vi "ReadSlotsNode.vi"(8 "Error In":errorcluster, 11 "Multiplexer Node In":refnum<k20>) -> (0 "Error Out":errorcluster, 2 "Slots":T1[](array[typedef]), 3 "Multiplexer Node Out":refnum<k20>)   [LabVIEW 2012]
uses:
  SlotConfiguration.ctl
  BankConfiguration.ctl
  <vilib>/xml/NI_XML.lvlib
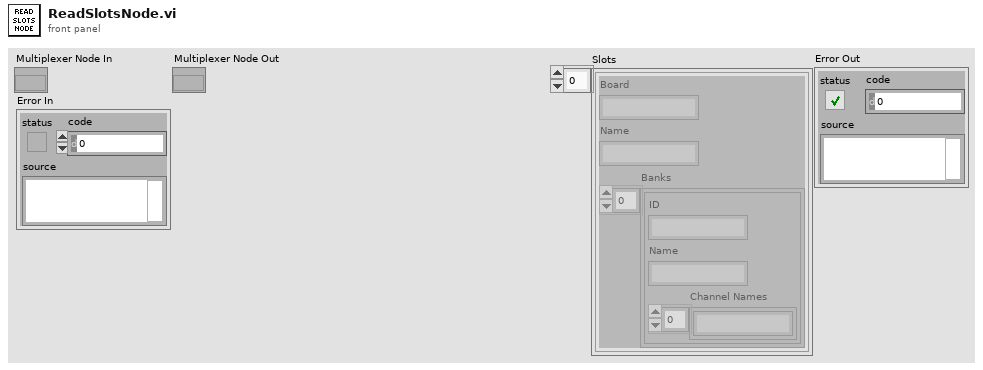
[diagram p1: front panel]
types:
  T1 = typedef "SlotConfiguration.ctl" = cluster{"Board":string, "Name":string, "Banks":T2[]}
  T2 = typedef "BankConfiguration.ctl" = cluster{"ID":string, "Name":string, "Channel Names":string[]}
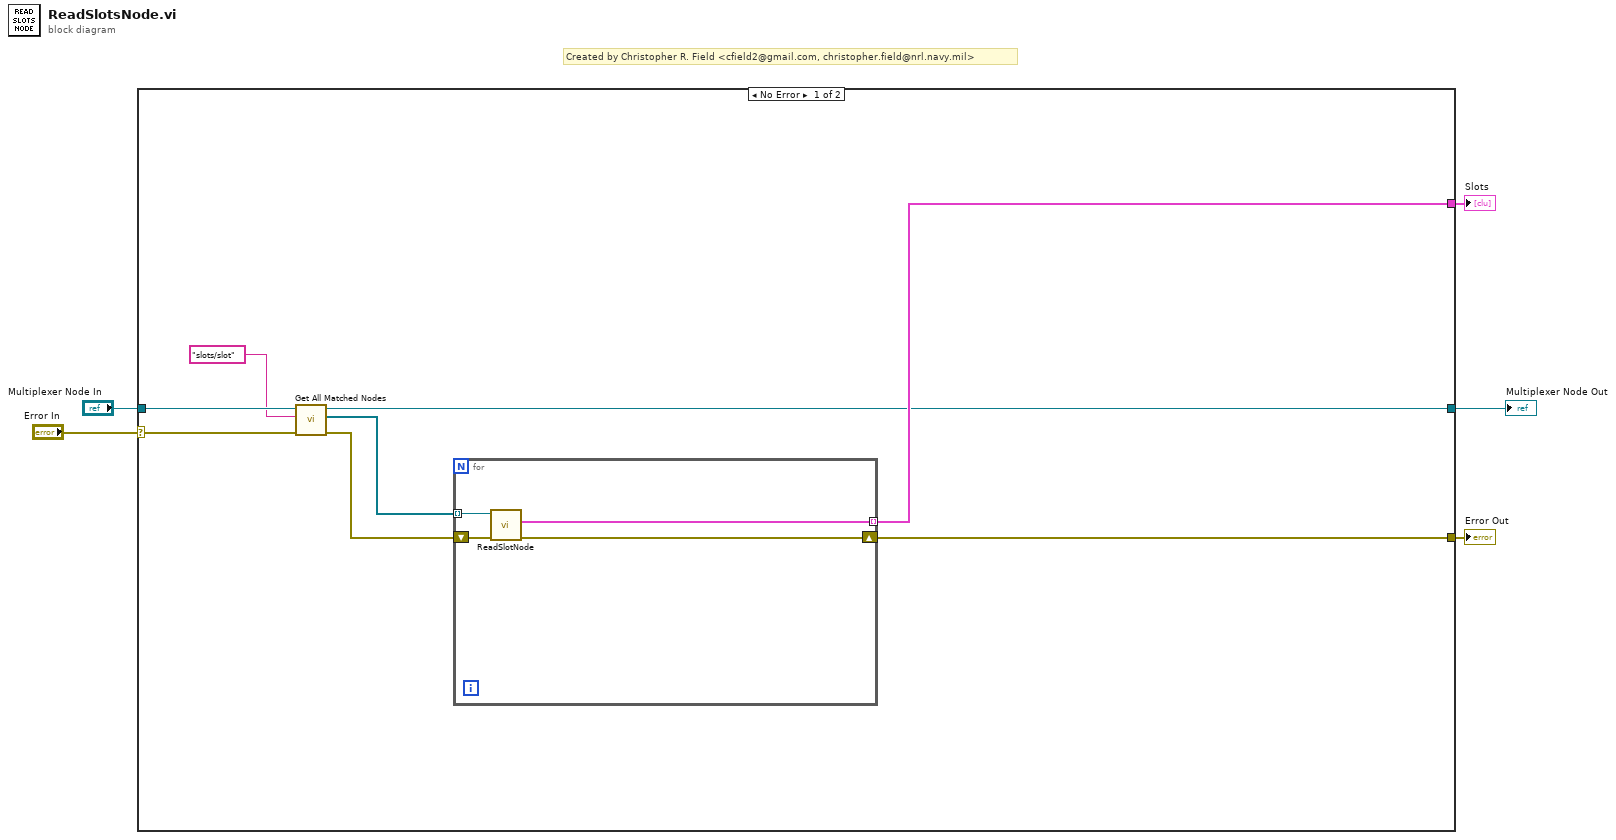
[diagram p0: block diagram]
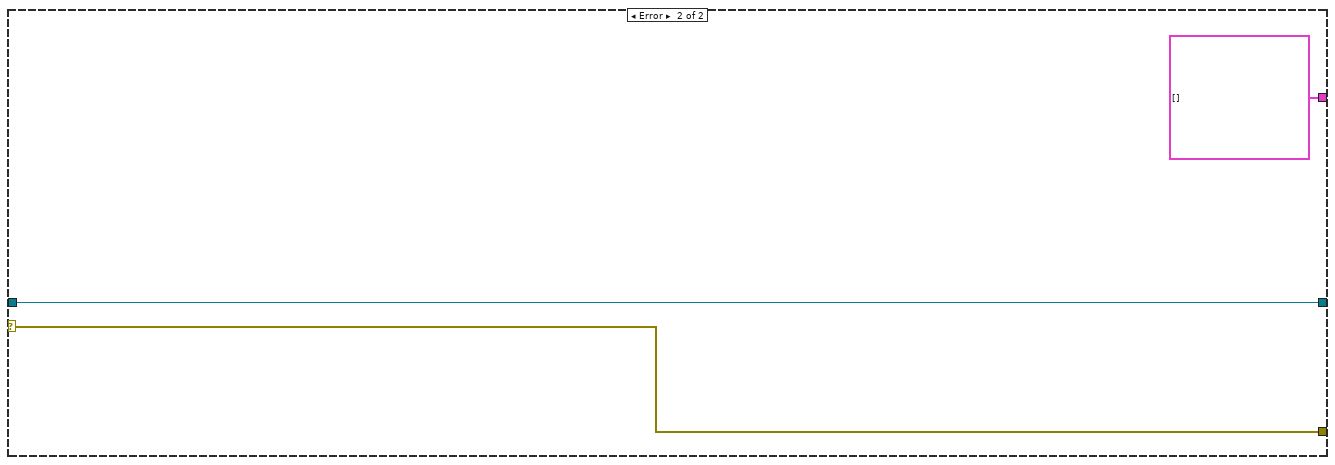
[diagram p2: hidden frame]
diagram:
  # "Created by Christopher R. Field <cfield2@gmail.com, christopher.field@nrl.navy.mil>"
  n1 = case shown="No Error" "Error In" {
    selector: "Error In" -> [w12 w19]
    tunnel: "Multiplexer Node In" -> [w13 w20]
    tunnel: [w8 T1[] []] -> w3
    tunnel: [w7 w20] -> w2
    tunnel: [w6 w19] -> w1
    frame No Error {
      n2 = call <vilib>:"Get All Matched Nodes.vi"("error in (no error)"=w12, "XPath expression"="slots/slot", "node in"=w13) -> ("error out"=w9:errorcluster, "node result array"=w10:refnum<k20>[], "node out"=w7:refnum<k20>)  [unwired: 6 in]
      n3 = for {
        tunnel: w10 -> [w17] mode=indexing
        shift-right: [w15] -> w6
        shift-left: w9 -> [w16]
        tunnel: [w14] -> w8 mode=indexing
        n4 = call "ReadSlotNode.vi"("Error In"=w16, "Slot Node In"=w17) -> ("Error Out"=w15:errorcluster, "Slot Configuration"=w14:T1)  [unwired: 7 in, 1 out]
      }
    }
    frame Error {
    }
  }
  "Slots" <- w3
  "Multiplexer Node Out" <- w2
  "Error Out" <- w1
